vi "DUAL GAUGE-Convert2Float.vi"(7 "W/R [W: Int in; Str out ]":bool, 9 "Eng2 in":dbl format="%.3f", 10 "Eng1 in":dbl format="%.3f", 11 "String in":string) -> (1 "Eng2 out":dbl format="%.3f", 2 "Eng1 out":dbl format="%.3f", 3 "String out":string)   [LabVIEW 2013, in "Dual Gauge.lvlib"]
uses:
  Dual Gauge.lvlib
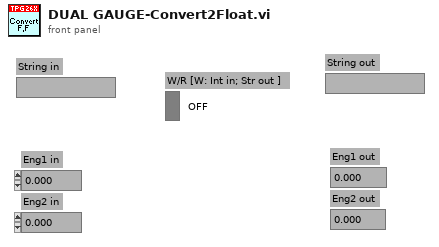
[diagram p1: front panel]
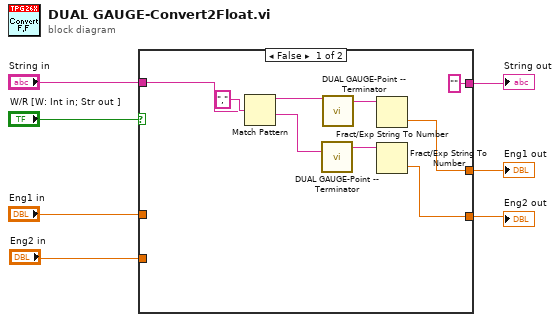
[diagram p0: block diagram]
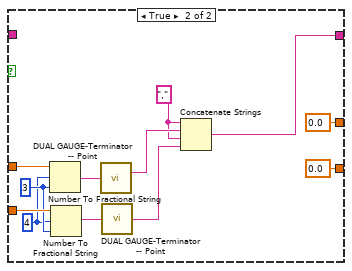
[diagram p2: hidden frame]
diagram:
  n1 = case shown="False" "W/R [W: Int in; Str out ]" {
    tunnel: "Eng1 in" -> [_ w28]
    tunnel: "Eng2 in" -> [_ w27]
    tunnel: ["" w22] -> w4
    tunnel: "String in" -> [w15 _]
    tunnel: [w12 0.0] -> w2
    tunnel: [w11 0.0] -> w1
    frame False {
      n2 = Match Pattern(string=w15, regular expression=",") -> (before substring=w9:string, after substring=w8:string)  [unwired: 1 in, 2 out]
      n3 = call "DUAL GAUGE-Point -- Terminator.vi"("Eingangstring"=w8) -> ("Ausgangstring"=w13:string)
      n4 = call "DUAL GAUGE-Point -- Terminator.vi"("Eingangstring"=w9) -> ("Ausgangstring"=w14:string)
      n5 = Fract/Exp String To Number(string=w14) -> (number=w11:dbl)  [unwired: 3 in, 1 out]
      n6 = Fract/Exp String To Number(string=w13) -> (number=w12:dbl)  [unwired: 3 in, 1 out]
    }
    frame True {
      w18 = i16 4 ("width (-)")
      w19 = i16 3 ("width (-)")
      w17 = ","
      n7 = Number To Fractional String(number=w28, width (-)=w18, precision (6)=w19) -> (F-format string=w26:string)  [unwired: 1 in]
      n8 = Number To Fractional String(number=w27, width (-)=w18, precision (6)=w19) -> (F-format string=w25:string)  [unwired: 1 in]
      n9 = call "DUAL GAUGE-Terminator -- Point.vi"("Eingangstring"=w26) -> ("Ausgangstring"=w24:string)
      n10 = call "DUAL GAUGE-Terminator -- Point.vi"("Eingangstring"=w25) -> ("Ausgangstring"=w23:string)
      n11 = Concatenate Strings(w17, w24, w17, w23) -> (w22:string)
    }
  }
  "String out" <- w4
  "Eng1 out" <- w1
  "Eng2 out" <- w2
